vi "03-和tsmaster配合演示接收报文.vi"() -> ()   [LabVIEW 2015]
panel:
  in  "GSINXTGP":u8
  in  "actual_toq":dbl(knob) scale=-280.0..300.0
  in  "rotate_speed":dbl(knob) scale=-11000.0..12000.0
  in  "停止":bool
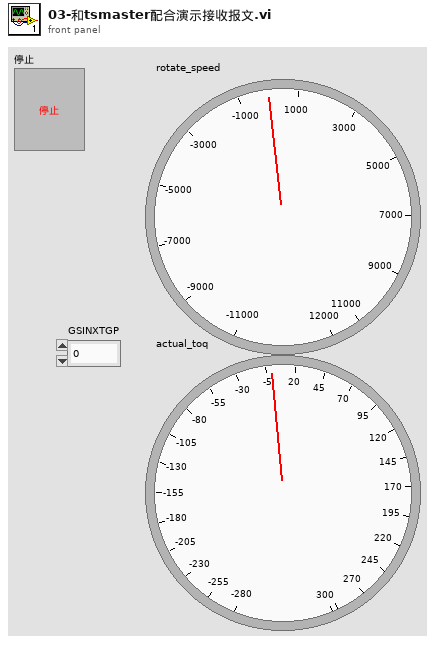
[diagram p1: front panel]
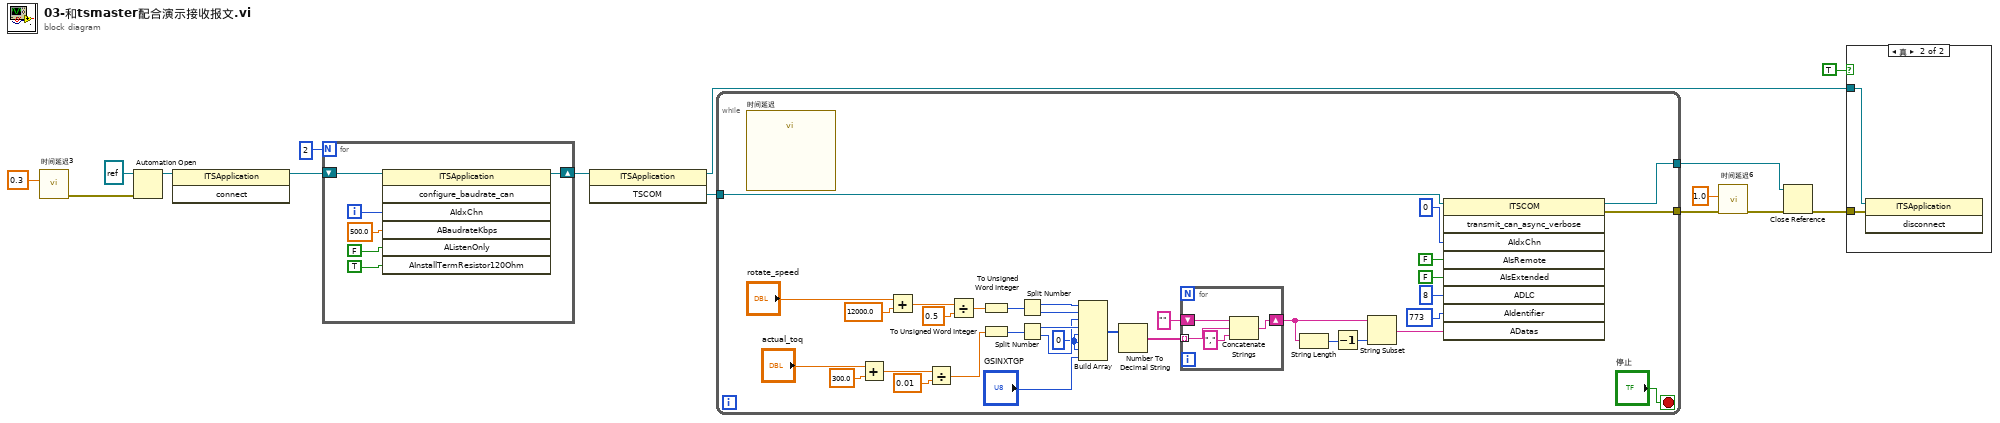
[diagram p0: block diagram]
diagram:
  n1 = call "时间延迟3"("Delay Time (s)"=0.3) -> ("error out"=w13:errorcluster)  [unwired: 10 in]
  n2 = Automation Open(error in (no error)=w13, Automation Refnum=refnum<k7> refnum ("TSMaster.ITSApplication")) -> (Automation Refnum=w7:refnum<k7>)  [unwired: 2 in, 1 out]
  n3 = invoke on="调用节点" class="ITSApplication" method="connect"(reference=w7) -> (reference out=w5:refnum<k7>)  [unwired: 2 in, 2 out]
  n4 = for {
    N: 2 -> [_]
    shift-right: [w20] -> w4
    shift-left: w5 -> [w21]
    i -> [w16]
    n5 = invoke on="调用节点" class="ITSApplication" method="configure_baudrate_can"(reference=w21, "AIdxChn"=w16, "ABaudrateKbps"=sgl 500.0, "AListenOnly"=FALSE, "AInstallTermResistor120Ohm"=TRUE) -> (reference out=w20:refnum<k7>)  [unwired: 2 in, 6 out]
  }
  n6 = invoke on="调用节点" class="ITSApplication" method="TSCOM"(reference=w4) -> (reference out=w9:refnum<k7>, "TSCOM"=w11:refnum<k7>)  [unwired: 2 in, 1 out]
  n7 = while {
    tunnel: w11 -> [w50]
    tunnel: [w49] -> w10
    tunnel: [w24] -> w3
    stop <- "停止" stop-if-true
    w26 = u8 0 ("元素")
    n8 = call "时间延迟"() -> ()  [unwired: 11 in, 1 out]
    n9 = Add(x="actual_toq", y=300.0) -> (x+y=w33:dbl)
    n10 = Add(x="rotate_speed", y=12000.0) -> (x+y=w40:dbl)
    n11 = Divide(x=w33, y=0.01) -> (x/y=w31:dbl)
    n12 = Divide(x=w40, y=0.5) -> (x/y=w38:dbl)
    n13 = To Unsigned Word Integer(number=w38) -> (unsigned 16bit integer=w37:u16)
    n14 = To Unsigned Word Integer(number=w31) -> (unsigned 16bit integer=w30:u16)
    n15 = Split Number(x=w37) -> (hi(x)=w36:u8, lo(x)=w35:u8)
    n16 = Split Number(x=w30) -> (hi(x)=w28:u8, lo(x)=w27:u8)
    n17 = Build Array(w36, w35, w27, w28, w26, w26, w26, "GSINXTGP") -> (w25:u8[])
    n18 = Number To Decimal String(number=w25) -> (decimal integer string=w47:string[])  [unwired: 1 in]
    n19 = for {
      tunnel: w47 -> [w58] mode=indexing
      shift-right: [w56] -> w45
      shift-left: "" -> [w59]
      n20 = Concatenate Strings(w59, w58, "," ("分隔符(Tab)")) -> (w56:string)
    }
    n21 = String Length(string=w45) -> (length=w46:i32)
    n22 = Decrement(x=w46) -> (x-1=w44:i32)
    n23 = String Subset(string=w45, length (rest)=w44) -> (substring=w43:string)  [unwired: 1 in]
    n24 = invoke on="调用节点" class="ITSCOM" method="transmit_can_async_verbose"(reference=w50, "AIdxChn"=0, "AIsRemote"=FALSE, "AIsExtended"=FALSE, "ADLC"=8, "AIdentifier"=773, "ADatas"=w43) -> (reference out=w24:refnum<k7>, error out=w49:errorcluster)  [unwired: 2 in, 7 out]
  }
  n25 = call "时间延迟6"("error in (no error)"=w10, "Delay Time (s)"=1.0) -> ("error out"=w2:errorcluster)  [unwired: 9 in]
  n26 = Close Reference(reference=w3, error in (no error)=w2) -> (error out=w1:errorcluster)
  n27 = case shown="真" TRUE {
    tunnel: w9 -> [_ w61]
    tunnel: w1 -> [_ w60]
    frame False {
    }
    frame True {
      n28 = invoke on="调用节点" class="ITSApplication" method="disconnect"(reference=w61, error in=w60) -> ()  [unwired: 1 in, 3 out]
    }
  }
